vi "test All Verifies With Labels.vi"(8 "error in":errorcluster, 11 "LUnit Test Case In":refnum<class "Test Case.lvclass">) -> (0 "error out":errorcluster, 3 "LUnit Test Case Out":refnum<class "Test Case.lvclass">)   [LabVIEW 2020, in "LUnit Extensions Tests.lvclass"]
uses:
  LUnit Extensions Tests.lvclass
  <vilib>/Astemes/LUnit/Test Case.lvclass
  Source/Approval Tests/Options/Options.lvclass/Options.ctl
  Source/Approval Tests/Naming Data/Naming Data.lvclass/Naming Data.ctl
  <vilib>/Astemes/LUnit/Test Case.lvclass/Test Case.ctl
  Source/Approval Tests/Options/Options.lvclass
  Source/Approval Tests/Scrubber/Scrubber.lvclass
  Source/Approval Tests/Namer/Namer.lvclass
  Source/Approval Tests/Naming Data/Naming Data.lvclass
  Source/Approval Tests/Reporter/Reporter.lvclass
  Source/Approval Tests/Text Comparator/Text Comparator.lvclass
  b408234e-25e8-47f8-b56b-8bcce1a32757.vi
  Source/Extensions/LUnit.Extension/LUnit.Extension.lvlib
  8ed6e648-6826-3fe0-2e6d-afd117c6e23f.vi
  4dde5500-32e6-3fd8-8833-a45ce68cea3f.vi
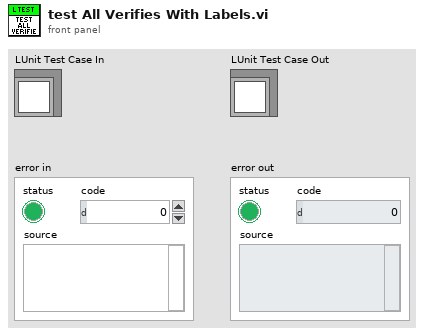
[diagram p1: front panel]
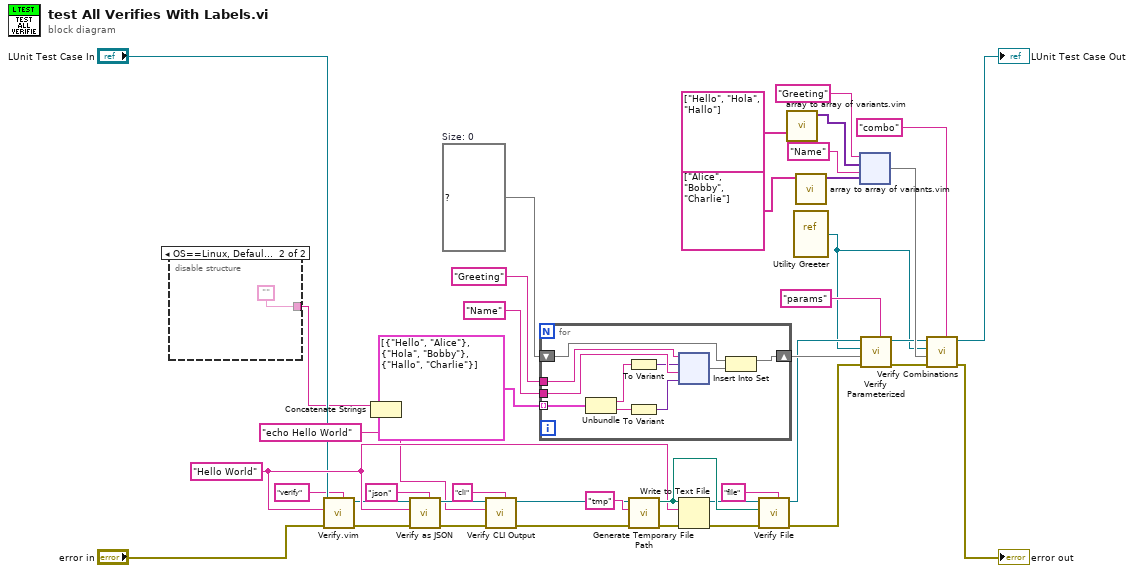
[diagram p0: block diagram]
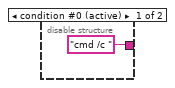
[diagram p2: hidden frame]
diagram:
  w31 = set{map{string, variant}} {}  # Size: 0
  w22 = "Hello World"
  n1 = disable-structure shown="OS==Linux, Default" {
    disable-tunnel: ["cmd /c " ""] -> w3
    frame condition #0 (active) {
    }
    frame condition #1 {
    }
  }
  n2 = call "Verify.vim"("Label"="verify", "error in"="error in", "Test Data"=w22, "LUnit Test Case In"="LUnit Test Case In") -> ("error out"=w41:errorcluster, "LUnit Test Case Out"=w20:refnum<class "Test Case.lvclass">)  [unwired: 6 in]
  n3 = Concatenate Strings(w3, "echo Hello World" ("string")) -> (w4:string)
  n4 = call "Verify as JSON.vi"("Label"="json", "error in"=w41, "Anything"=w22, "LUnit Test Case In"=w20) -> ("error out"=w40:errorcluster, "LUnit Test Case Out"=w19:refnum<class "Test Case.lvclass">)  [unwired: 6 in]
  n5 = call "Verify CLI Output.vi"("Label"="cli", "error in"=w40, "command line"=w4, "LUnit Test Case In"=w19) -> ("error out"=w37:errorcluster, "LUnit Test Case Out"=w18:refnum<class "Test Case.lvclass">)  [unwired: 6 in]
  n6 = for {
    tunnel: "Greeting" -> [w53]
    tunnel: cluster{string, string}[] [{"Hello", "Alice"}, {"Hola", "Bobby"}, {"Hallo", "Charlie"}] -> [w51] mode=indexing
    tunnel: "Name" -> [w52]
    shift-right: [w45] -> w32
    shift-left: w31 -> [w44]
    n7 = Unbundle(w51) -> (w50:string, w49:string)
    n8 = To Variant(anything=w50) -> (Variant=w47:variant)
    n9 = To Variant(anything=w49) -> (Variant=w46:variant)
    n10 = node ("Build Map")(w53, w47, w52, w46) -> (w48:map{string, variant})
    n11 = Insert Into Set(10:w48, 11:w44) -> (3:w45:set{map{string, variant}})  [unwired: 1 out]
  }
  n12 = call <vilib>:"Generate Temporary File Path.vi"("error in (no error)"=w37, "Temporary File Extension (tmp)"="tmp") -> ("error out"=w36:errorcluster, "Unique Temporary File Path"=w23:path)  [unwired: 8 in]
  n13 = Write to Text File(file (use dialog)=w23, text=w22, error in=w36) -> (error out=w35:errorcluster)  [unwired: 1 in, 2 out]
  n14 = call "Verify File.vi"("Label"="file", "error in"=w35, "path to file"=w23, "LUnit Test Case In"=w18) -> ("error out"=w39:errorcluster, "LUnit Test Case Out"=w17:refnum<class "Test Case.lvclass">)  [unwired: 6 in]
  n15 = call "array to array of variants.vim"("Array in"=string[] ["Hello", "Hola", "Hallo"]) -> ("Array out"=w7:variant[])  [unwired: 10 in]
  n16 = vi-ref "Utility Greeter.vi"() -> (w1:refnum<vi>)
  n17 = call "array to array of variants.vim"("Array in"=string[] ["Alice", "Bobby", "Charlie"]) -> ("Array out"=w5:variant[])  [unwired: 10 in]
  n18 = node ("Build Map")("Greeting" ("key"), w7, "Name" ("key"), w5) -> (w27:map{string, variant[]})
  n19 = call "Verify Parameterized.vi"("Label"="params", "error in"=w39, "Set of ctl label -> value var"=w32, "VI in"=w1, "LUnit Test Case In"=w17) -> ("error out"=w38:errorcluster, "LUnit Test Case Out"=w16:refnum<class "Test Case.lvclass">)  [unwired: 5 in]
  n20 = call "Verify Combinations.vi"("Label"="combo", "error in"=w38, "ctl label -> value var[]"=w27, "VI in"=w1, "LUnit Test Case In"=w16) -> ("error out"=→"error out":errorcluster, "LUnit Test Case Out"=→"LUnit Test Case Out":refnum<class "Test Case.lvclass">)  [unwired: 5 in]
